vi "Shooter Global.vi"() -> ()   [LabVIEW 2011]
uses:
  Shared/Shooter Control Mode.ctl
panel:
  in  "Shooter Speed Enumerated Type":T1=enum."Off"
  out "Internal Mode":T2(ring)
  in  "Shooter Mode":T3(ring)
  out "Motor Speed":dbl
  out "Current RPM":dbl
  in  "Set Motor Speed":dbl caption="(Open Loop Control)"
  in  "Set RPM":dbl caption="(Closed Loop Control)"
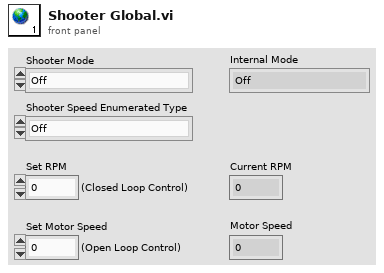
[diagram p1: front panel]
types:
  T1 = typedef "Shooter Control Mode.ctl" = enum16{"Key", "Mid Field", "Backfield", "Topspin", "Open Loop Control", "Off"}
  T2 = enum16{"Off", "Open Loop Control", "Closed Loop", "Top Spin", "Wait for Spindown"}
  T3 = enum16{"Off", "Open Loop Control", "Closed Loop Control", "Top Spin"}
diagram:
